vi "Get Parameters Configuration File Path.vi"(8 "error in":errorcluster, 11 "custom device ref":T1 format="%.0x") -> (0 "error out":errorcluster, 2 "path":path, 3 "custom device ref out":T1 format="%.0x")   [LabVIEW 2020, in "ARINC 429 Scripting.lvlib"]
uses:
  ARINC 429 Scripting.lvlib
  <vilib>/NI VeriStand/Custom Device API/Custom Device Item Ref.ctl
  Ballard/Constants.vi
  <vilib>/NI VeriStand/Custom Device API/Get Item Property (Path).vi
  Ballard/Ballard ARINC 429 Scripting.lvlib
  <vilib>/NI VeriStand/Custom Device API/Custom Device API.lvlib
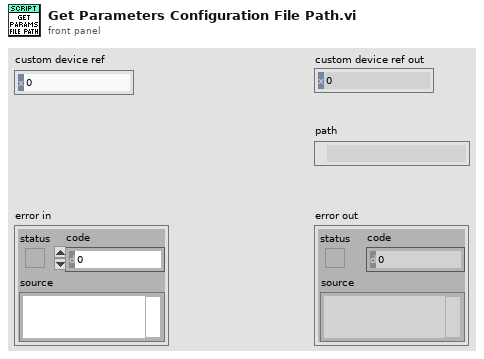
[diagram p1: front panel]
types:
  T1 = typedef "Custom Device API.lvlib/Custom Device Item Ref.ctl" = u64
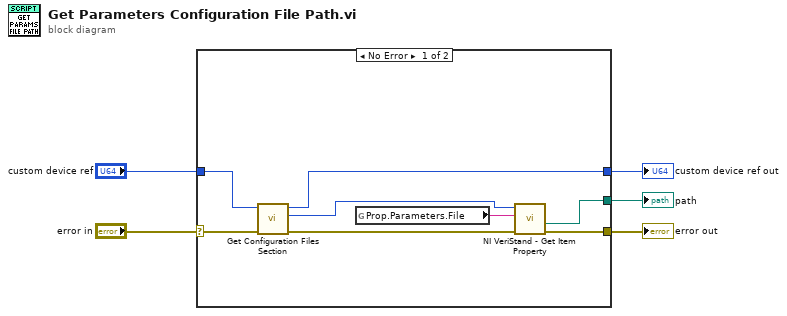
[diagram p0: block diagram]
diagram:
  n1 = case shown="No Error" "error in" {
    selector: "error in" -> [w8 w15]
    tunnel: "custom device ref" -> [w9 w14]
    tunnel: [w11 w15] -> w4
    tunnel: [w6 w14] -> w2
    tunnel: [w12 _] -> w1
    frame No Error {
      n2 = call "Get Configuration Files Section.vi"("error in"=w8, "Custom device Ref"=w9) -> ("error out"=w7:errorcluster, "Configuration files Ref"=w10:T1, "Custom device Ref out"=w6:T1)  [unwired: 7 in]
      n3 = global read "Constants.vi" "Prop.Parameters.File"() -> (w13:string)
      n4 = call-poly <vilib>:"NI VeriStand - Get Item Property.vi"("error in (no error)"=w7, "Property Name"=w13, "Item Ref in"=w10) -> ("error out"=w11:errorcluster, "Value"=w12:path)  [unwired: 5 in, 2 out]
    }
    frame Error {
    }
  }
  "error out" <- w4
  "path" <- w1
  "custom device ref out" <- w2
